vi "Save-LVDR-Data.vi"() -> ()   [LabVIEW 2011]
panel:
  out "FileString":string
  in  "EPOCH":dbl format="%.2f"
  out "File Path":path
  in  "Directory":path
  in  "Data":dbl[](array[numeric])
  in  "DEC":dbl format="%<%H:%M:%S%1u>t"
  in  "HA":dbl format="%<%H:%M:%S%1u>t"
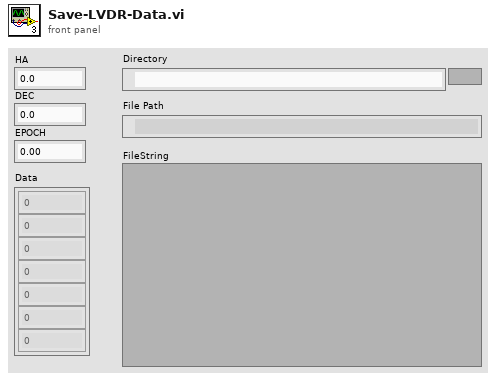
[diagram p1: front panel]
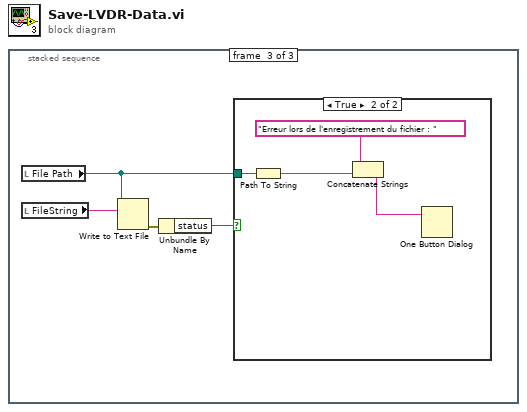
[diagram p0: block diagram]
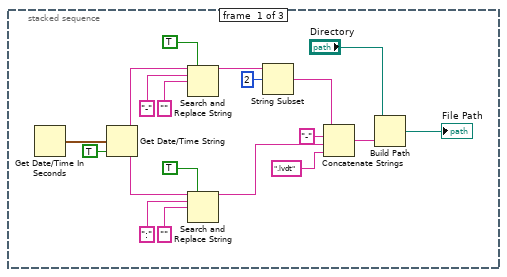
[diagram p2: hidden frame]
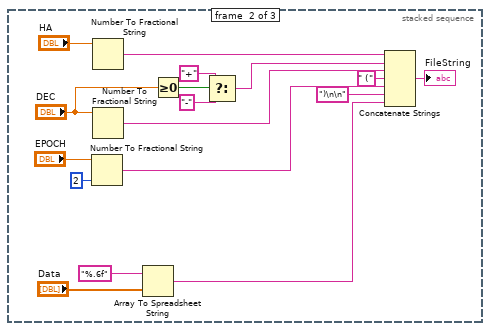
[diagram p3: hidden frame]
diagram:
  n1 = stacked-sequence {
    frame #0 {
      n2 = Get Date/Time In Seconds() -> (seconds since 1Jan1904=w19:timestamp)
      n3 = Get Date/Time String(seconds (now)=w19, want seconds? (F)=TRUE) -> (date string=w17:string, time string=w9:string)  [unwired: 1 in]
      n4 = Search and Replace String(replace all?=TRUE ("replace all? (F)"), input string=w17, search string="-", replace string="" ("replace string (\"\")")) -> (result string=w13:string)  [unwired: 4 in, 3 out]
      n5 = Search and Replace String(replace all?=TRUE ("replace all? (F)"), input string=w9, search string=":", replace string="" ("replace string (\"\")")) -> (result string=w6:string)  [unwired: 4 in, 3 out]
      n6 = String Subset(string=w13, offset (0)=2) -> (substring=w7:string)  [unwired: 1 in]
      n7 = Concatenate Strings(w7, "-" ("string"), w6, ".lvdt" ("string")) -> (w3:string)
      n8 = Build Path(base path="Directory", name or relative path=w3) -> (appended path=→"File Path":path)
    }
    frame #1 {
      n9 = Number To Fractional String(number="EPOCH", precision (6)=i16 2) -> (F-format string=w24:string)  [unwired: 2 in]
      n10 = Number To Fractional String(number="HA") -> (F-format string=w33:string)  [unwired: 3 in]
      n11 = Number To Fractional String(number="DEC") -> (F-format string=w32:string)  [unwired: 3 in]
      n12 = Array To Spreadsheet String(array="Data", 3:"%.6f") -> (spreadsheet string=w22:string)  [unwired: 1 in]
      n13 = Greater Or Equal To 0?(x="DEC") -> (x >= 0?=w31:bool)
      n14 = Select(t="+", s=w31, f="-") -> (s? t:f=w27:string)
      n15 = Concatenate Strings(w33, w27, w32, " (" ("string"), w24, ")\n\n" ("string"), w22) -> (→"FileString":string)
    }
    frame #2 {
      n16 = local read "File Path"() -> (w37:path)
      n17 = local read "FileString"() -> (w40:string)
      n18 = Write to Text File(file (use dialog)=w37, text=w40) -> (error out=w39:errorcluster)  [unwired: 2 in, 2 out]
      n19 = Unbundle By Name(w39) -> ("status"=w38:bool)
      n20 = case shown="True" w38 {
        tunnel: w37 -> [_ w44]
        frame False {
        }
        frame True {
          n21 = Path To String(path=w44) -> (string=w43:string)
          n22 = Concatenate Strings("Erreur lors de l'enregistrement du fichier : ", w43) -> (w41:string)
          n23 = One Button Dialog(message=w41) -> ()  [unwired: 1 in, 1 out]
        }
      }
    }
  }
